vi "get_python_library_path.vi"() -> (3 "Python library path":path)   [LabVIEW 2020]
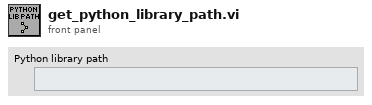
[diagram p1: front panel]
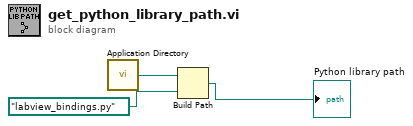
[diagram p0: block diagram]
diagram:
  n1 = call <vilib>:"Application Directory.vi"() -> ("Application Directory"=w1:path)
  n2 = Build Path(base path=w1, name or relative path=path "labview_bindings.py" ("module path")) -> (appended path=→"Python library path":path)
